vi "save DAQ configuration.vi"(8 "error in (no error)":errorcluster, 9 "Write Ini":bool, 10 "Read Ini":bool, 11 "Path":path=path "C:/Users/CWEDD/Documents/LabVIEW Data/Waterloo DAQ/config files/DAQ Setup Config.ini") -> (0 "error out":errorcluster)   [LabVIEW 2015]
uses:
  controls/Aux Sensor.ctl
  controls/MCC DAQ Setup.ctl
  <vilib>/Utility/config.llb/NI_LVConfig.lvlib
  <vilib>/Utility/VariantDataType/VariantType.lvlib
panel:
  out "delimited string":string
  in  "MCC USB-DAQ Setup":T1={"Device Name in InstaCal"="Dev0", "Omega Pressure Sensor"={"DAQ Channel"=2.0, "Output Voltage Range"=1, "Enabled"=TRUE, "Description"="Uphole Pressure"}, "McMillian 102 Flowmeter"={"DAQ Channel"=11.0, "Output Voltage Range"=1, "Enabled"=TRUE, "Description"="Flow"}, "DHT Pressure Sensor"={"DAQ Channel"=3.0, "Output Voltage Range"=1, "Enabled"=TRUE, "Description"="Downhole Pressure"}, "Top String Pot"={"DAQ Channel"=0.0, "Output Voltage Range"=0, "Enabled"=TRUE, "Description"="Top String Pot"}, "String Pot Signal"={"DAQ Channel"=1.0, "Output Voltage Range"=0, "Enabled"=TRUE, "Description"="String Pot"}, "Aux Sensor 1"={"DAQ Channel"=5.0, "Output Voltage Range"=1, "Enabled"=FALSE, "Description"="Aux 1"}, "Aux Sensor 2"={"DAQ Channel"=6.0, "Output Voltage Range"=1, "Enabled"=FALSE, "Description"="Aux 2"}, "Aux Sensor 3"={"DAQ Channel"=7.0, "Output Voltage Range"=1, "Enabled"=TRUE, "Description"="Aux 3"}, "Aux Sensor 4"={"DAQ Channel"=15.0, "Output Voltage Range"=1, "Enabled"=TRUE, "Description"="Aux 4"}, "Voltage Monitor"={"DAQ Channel"=8.0, "Output Voltage Range"=0, "Enabled"=TRUE, "Description"="9V Monitor"}} {"Voltage Monitor"."Output Voltage Range" items=["+/-10 V Range", "+/-5 V Range", "+/-2.5V Range", "+/-1.25 V Range", "+/-0.625 V Range", "+/-0.3125 V Range", "+/-0.1562V Range", "+/-0.078125 V Range"]; "Aux Sensor 4"."Output Voltage Range" items=["+/-10 V Range", "+/-5 V Range", "+/-2.5V Range", "+/-1.25 V Range", "+/-0.625 V Range", "+/-0.3125 V Range", "+/-0.1562V Range", "+/-0.078125 V Range"]; "Aux Sensor 3"."Output Voltage Range" items=["+/-10 V Range", "+/-5 V Range", "+/-2.5V Range", "+/-1.25 V Range", "+/-0.625 V Range", "+/-0.3125 V Range", "+/-0.1562V Range", "+/-0.078125 V Range"]; "Aux Sensor 2"."Output Voltage Range" items=["+/-10 V Range", "+/-5 V Range", "+/-2.5V Range", "+/-1.25 V Range", "+/-0.625 V Range", "+/-0.3125 V Range", "+/-0.1562V Range", "+/-0.078125 V Range"]; "Aux Sensor 1"."Output Voltage Range" items=["+/-10 V Range", "+/-5 V Range", "+/-2.5V Range", "+/-1.25 V Range", "+/-0.625 V Range", "+/-0.3125 V Range", "+/-0.1562V Range", "+/-0.078125 V Range"]; "String Pot Signal"."Output Voltage Range" items=["+/-10 V Range", "+/-5 V Range", "+/-2.5V Range", "+/-1.25 V Range", "+/-0.625 V Range", "+/-0.3125 V Range", "+/-0.1562V Range", "+/-0.078125 V Range"]; "Top String Pot"."Output Voltage Range" items=["+/-10 V Range", "+/-5 V Range", "+/-2.5V Range", "+/-1.25 V Range", "+/-0.625 V Range", "+/-0.3125 V Range", "+/-0.1562V Range", "+/-0.078125 V Range"]; "DHT Pressure Sensor"."Output Voltage Range" items=["+/-10 V Range", "+/-5 V Range", "+/-2.5V Range", "+/-1.25 V Range", "+/-0.625 V Range", "+/-0.3125 V Range", "+/-0.1562V Range", "+/-0.078125 V Range"]; "McMillian 102 Flowmeter"."Output Voltage Range" items=["+/-10 V Range", "+/-5 V Range", "+/-2.5V Range", "+/-1.25 V Range", "+/-0.625 V Range", "+/-0.3125 V Range", "+/-0.1562V Range", "+/-0.078125 V Range"]; "Omega Pressure Sensor"."Output Voltage Range" items=["+/-10 V Range", "+/-5 V Range", "+/-2.5V Range", "+/-1.25 V Range", "+/-0.625 V Range", "+/-0.3125 V Range", "+/-0.1562V Range", "+/-0.078125 V Range"]}
  out "Array":string[](array[string])
  in  "Sensor":T2={"DAQ Channel"=7.0, "Output Voltage Range"=0, "Enabled"=TRUE, "Description"=""} {"Output Voltage Range" items=["+/-10 V Range", "+/-5 V Range", "+/-2.5V Range", "+/-1.25 V Range", "+/-0.625 V Range", "+/-0.3125 V Range", "+/-0.1562V Range", "+/-0.078125 V Range"]}
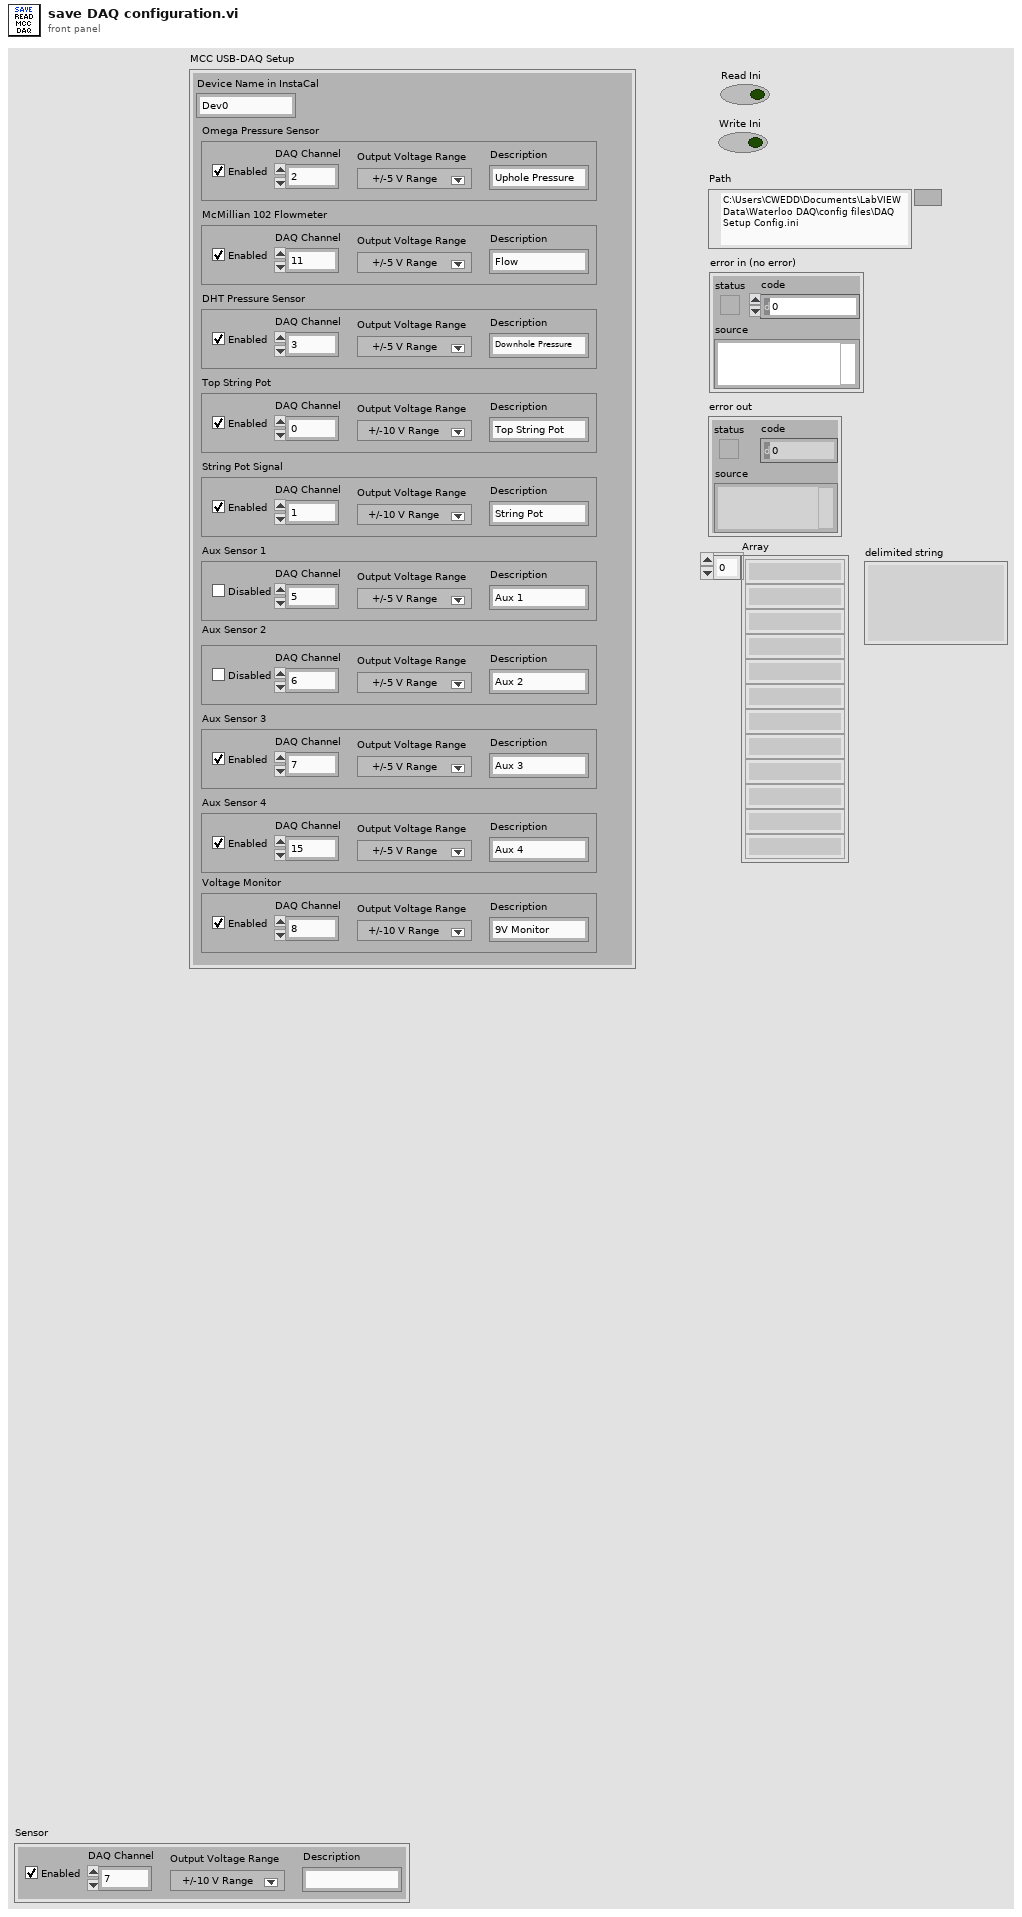
[diagram p1: front panel]
types:
  T1 = typedef "MCC DAQ Setup.ctl" = cluster{"Device Name in InstaCal":string, "Omega Pressure Sensor":T2, "McMillian 102 Flowmeter":T2, "DHT Pressure Sensor":T2, "Top String Pot":T2, "String Pot Signal":T2, "Aux Sensor 1":T2, "Aux Sensor 2":T2, "Aux Sensor 3":T2, "Aux Sensor 4":T2, "Voltage Monitor":T2}
  T2 = typedef "Aux Sensor.ctl" = cluster{"DAQ Channel":dbl, "Output Voltage Range":u16, "Enabled":bool, "Description":string}
  T3 = typedef "NI_LVConfig.lvlib/Config Data RefNum.ctl" = refnum<k1>
  T4 = typedef "VariantType.lvlib/TypedefInfo.ctl" = cluster{"Name":string, "Timestamp":u32}
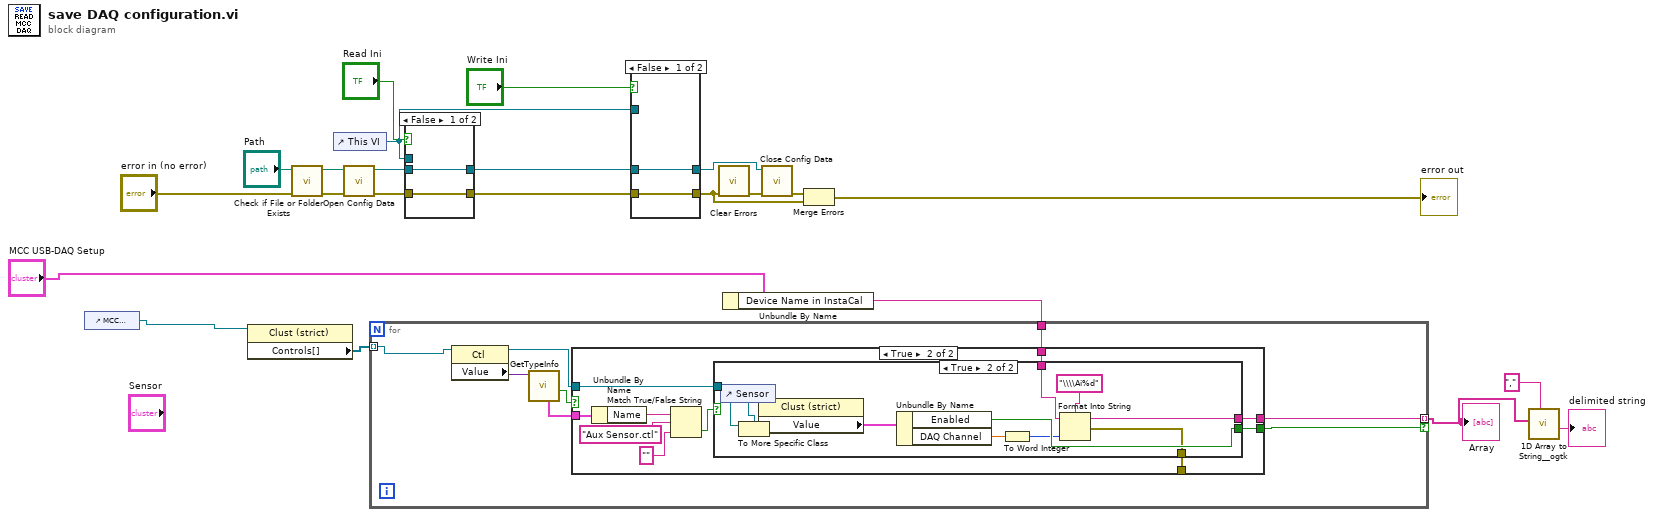
[diagram p0: block diagram]
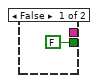
[diagram p2: hidden frame]
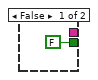
[diagram p3: hidden frame]
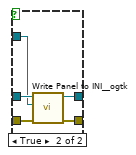
[diagram p4: hidden frame]
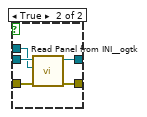
[diagram p5: hidden frame]
diagram:
  n1 = control-ref of="MCC USB-DAQ Setup"() -> (w4:refnum<vi>)
  n2 = property class="Clust (strict)"(reference=w4) -> ("Controls[]"=w7:refnum<vi>[])  [unwired: 1 in, 2 out]
  n3 = call <vilib>:"Check if File or Folder Exists.vi"("error in (no error)"="error in (no error)", "path"="Path") -> ("error out"=w19:errorcluster, "dup path"=w20:path)  [unwired: 7 in, 1 out]
  n4 = control-ref of="This VI"() -> (w11:refnum<vi>)
  n5 = call <vilib>:"Open Config Data.vi"("error in (no error)"=w19, "configuration file path"=w20) -> ("error out"=w17:errorcluster, "refnum"=w18:T3)  [unwired: 7 in, 1 out]
  n6 = case shown="False" "Read Ini" {
    tunnel: w18 -> [w25 w30]
    tunnel: w17 -> [w24 w29]
    tunnel: w11 -> [_ w28]
    tunnel: [w24 w27] -> w12
    tunnel: [w25 w26] -> w13
    frame False {
    }
    frame True {
      n7 = call <userlib>:"Read Panel from INI__ogtk.vi"("error in (no error)"=w29, "VI ref"=w28, "refnum"=w30) -> ("error out"=w27:errorcluster, "refnum out"=w26:T3)  [unwired: 7 in]
    }
  }
  n8 = case shown="False" "Write Ini" {
    tunnel: w13 -> [w32 w37]
    tunnel: w12 -> [w31 w36]
    tunnel: w11 -> [_ w35]
    tunnel: [w32 w34] -> w10
    tunnel: [w31 w33] -> w9
    frame False {
    }
    frame True {
      n9 = call <userlib>:"Write Panel to INI__ogtk.vi"("error in (no error)"=w36, "VI ref"=w35, "refnum"=w37) -> ("error out"=w33:errorcluster, "refnum out"=w34:T3)  [unwired: 7 in]
    }
  }
  n10 = call <vilib>:"Clear Errors.vi"("error in (no error)"=w9) -> ("error out"=w16:errorcluster)  [unwired: 5 in, 1 out]
  n11 = Unbundle By Name("MCC USB-DAQ Setup") -> ("Device Name in InstaCal"=w6:string)
  n12 = for {
    tunnel: w7 -> [w45] mode=indexing
    tunnel: w6 -> [w40]
    tunnel: [w39] -> w3 mode=indexing if=w38
    n13 = property class="Ctl"(reference=w45) -> (reference out=w41:refnum<vi>, "Value"=w44:variant)  [unwired: 1 in, 1 out]
    n14 = call <vilib>:"GetTypeInfo.vi"("Variant"=w44) -> ("HasTypedef"=w43:bool, "TypedefInfo"=w42:T4)  [unwired: 6 in, 3 out]
    n15 = case shown="True" w43 {
      tunnel: w42 -> [_ w56]
      tunnel: w41 -> [_ w52]
      tunnel: w40 -> [_ w51]
      tunnel: [_ w50] -> w39
      tunnel: [FALSE ("Enabled") w49] -> w38
      tunnel: [_ w47] -> _
      frame False {
      }
      frame True {
        n16 = Unbundle By Name(w56) -> ("Name"=w55:string)
        n17 = Match True/False String(2:"" ("false string"), 3:"Aux Sensor.ctl" ("true string"), 4:w55) -> (0:w53:bool)  [unwired: 1 out]
        n18 = case shown="True" w53 {
          tunnel: w52 -> [_ w68]
          tunnel: w51 -> [_ w64]
          tunnel: [_ w61] -> w50
          tunnel: [FALSE ("Enabled") w60] -> w49
          tunnel: [_ w58] -> w47
          frame False {
          }
          frame True {
            n19 = control-ref of="Sensor"() -> (w66:refnum<vi>)
            n20 = To More Specific Class(target class=w66, reference=w68) -> (specific class reference=w67:refnum<vi>)  [unwired: 1 in, 1 out]
            n21 = property class="Clust (strict)"(reference=w67) -> ("Value"=w65:T2)  [unwired: 1 in, 2 out]
            n22 = Unbundle By Name(w65) -> ("Enabled"=w60:bool, "DAQ Channel"=w62:dbl)
            n23 = To Word Integer(number=w62) -> (16bit integer=w59:i16)
            n24 = Format Into String(format string="\\\\Ai%d", initial string=w64, w59) -> (resulting string=w61:string, error out=w58:errorcluster)  [unwired: 1 in]
          }
        }
      }
    }
  }
  "Array" <- w3
  n25 = call <vilib>:"Close Config Data.vi"("error in (no error)"=w16, "refnum"=w10) -> ("error out"=w15:errorcluster)  [unwired: 8 in, 1 out]
  n26 = Merge Errors(w15, w9) -> (→"error out":errorcluster)
  n27 = call <userlib>:"1D Array to String__ogtk.vi"("delimiter (Tab)"=",", "Array of Strings"=w3) -> ("delimited string"=→"delimited string":string)  [unwired: 9 in]
